vi "main.vi"() -> ()   [LabVIEW 2016]
uses:
  Monochromator/Monochromator.lvclass
  MonoStateFactory/MonoStateFactory.lvclass
  ts_labview_tcp/TCPServer/TCPServer.lvclass
  C:/Users/aanania/Documents/ts_monochromator_windows/ts_labview_tcp/TCPCommunicator/TCPCommunicator.lvclass
  ts_labview_tcp/TCPComEvents/TCPComEvents.lvclass
  MonoCommunicator/MonoCommunicator.lvclass
  MonoPubSubData/MonoPubSubData.lvclass
  Typedefs/SWStatus.ctl
  Monochromator/Monochromator.lvclass/Monochromator.ctl
  MonoPubSubData/MonoPubSubData.lvclass/MonoPubSubData.ctl
  MonoCommunicator/MonoCommunicator.lvclass/MonoCommunicator.ctl
  ts_labview_tcp/TCPComEvents/TCPComEvents.lvclass/TCPComEvents.ctl
  ts_labview_tcp/TCPCommunicator/TCPCommunicator.lvclass/TCPCommunicator.ctl
  Monochromator/run.vi
  ts_labview_tcp/TCPSettings/TCPSettings.lvclass
  ts_labview_tcp/TCPCommunicator/TCPCommunicator.lvclass
panel:
  in  "Port":u16=50000
  in  "IP":string="127.0.0.1"
  in  "MonoID":string="Mono1"
  in  "Force Init":bool
  in  "UniqueID":string
  # "Mono Init"
  # "TCP Setting"
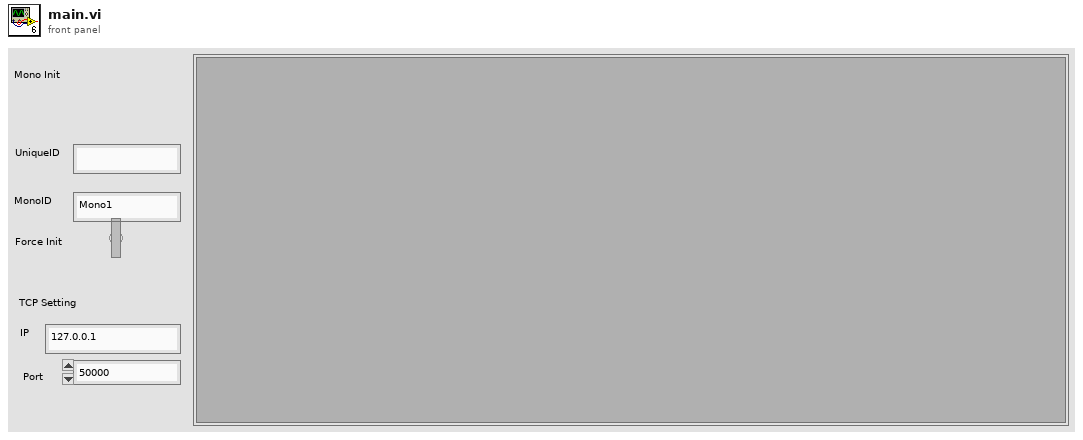
[diagram p1: front panel]
types:
  T1 = typedef "SWStatus.ctl" = enum16{"OfflineState", "ReadyState", "SettingUpState", "FaultState"}
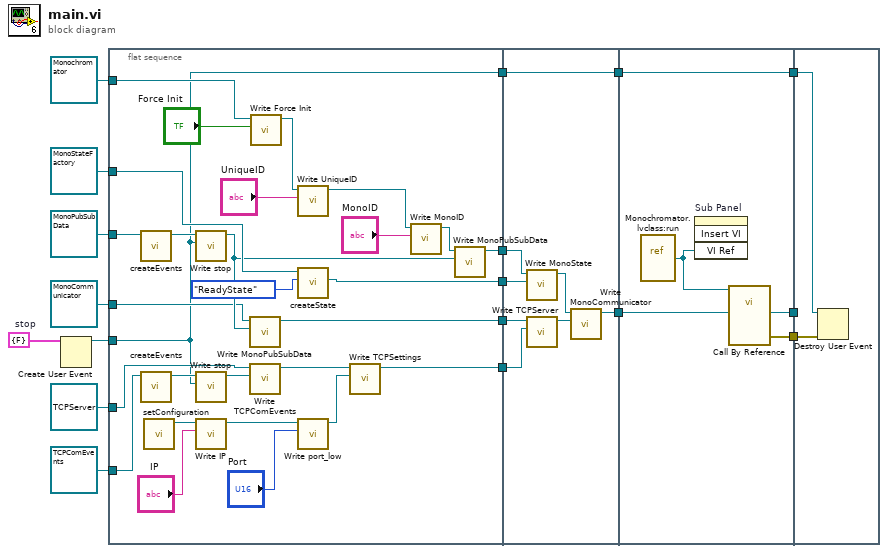
[diagram p0: block diagram]
diagram:
  w12 = cluster{"stop":bool} {"stop"=FALSE}  # stop
  n1 = Create User Event(user event datatype=w12) -> (user event=w11:refnum<user-event>)  [unwired: 1 in, 1 out]
  n2 = flat-sequence {
    tunnel: refnum<class "Monochromator.lvclass"> refnum ("Monochromator.lvclass") -> [w45]
    tunnel: [w32] -> w17
    tunnel: refnum<class "MonoStateFactory.lvclass"> refnum ("MonoStateFactory.lvclass") -> [w42]
    tunnel: [w40] -> w15
    tunnel: refnum<class "TCPComEvents.lvclass"> refnum ("TCPComEvents.lvclass") -> [w39]
    tunnel: refnum<class "TCPServer.lvclass"> refnum ("TCPServer.lvclass") -> [w37]
    tunnel: w11 -> [w27]
    tunnel: [w34] -> w10
    tunnel: refnum<class "MonoPubSubData.lvclass"> refnum ("MonoPubSubData.lvclass") -> [w33]
    tunnel: refnum<class "MonoCommunicator.lvclass"> refnum ("MonoCommunicator.lvclass") -> [w29]
    tunnel: [w28] -> w7
    tunnel: [w27] -> w3
    tunnel: w17 -> [w54]
    tunnel: w15 -> [w53]
    tunnel: w10 -> [w51]
    tunnel: w7 -> [w52]
    tunnel: [w48] -> w6
    tunnel: [w47] -> w4
    tunnel: w3 -> [w47]
    tunnel: w6 -> [w57]
    tunnel: [w59] -> w5
    tunnel: w4 -> [w59]
    tunnel: [w56] -> w2
    tunnel: [w55] -> w1
    tunnel: w5 -> [w61]
    tunnel: w2 -> [_]
    tunnel: w1 -> [w60]
    frame #0 {
      n3 = call "createEvents.vi"("MonoPubSubData in"=w33) -> ("MonoPubSubData out"=w31:refnum<class "MonoPubSubData.lvclass">)  [unwired: 9 in, 1 out]
      n4 = call "createEvents.vi"("TCPComEvents in"=w39) -> ("TCPComEvents out"=w38:refnum<class "TCPComEvents.lvclass">)  [unwired: 9 in, 1 out]
      n5 = call "setConfiguration.vi"() -> ("TCPSettings out"=w23:refnum<class "TCPSettings.lvclass">)  [unwired: 11 in]
      n6 = call "Write stop.vi"("stop"=w27, "MonoPubSubData in"=w31) -> ("MonoPubSubData out"=w30:refnum<class "MonoPubSubData.lvclass">)  [unwired: 8 in, 1 out]
      n7 = call "Write stop.vi"("stop"=w27, "TCPComEvents in"=w38) -> ("TCPComEvents out"=w36:refnum<class "TCPComEvents.lvclass">)  [unwired: 8 in, 1 out]
      n8 = call-dynamic "Write IP.vi"("IP"="IP", "TCPSettings in"=w23) -> ("TCPSettings out"=w21:refnum<class "TCPSettings.lvclass">)  [unwired: 8 in, 1 out]
      n9 = call "Write MonoPubSubData.vi"("MonoPubSubData.lvclass"=w30, "MonoCommunicator in"=w29) -> ("MonoCommunicator out"=w28:refnum<class "MonoCommunicator.lvclass">)  [unwired: 8 in, 1 out]
      n10 = call "Write TCPComEvents.vi"("TCPComEvents.lvclass"=w36, "TCPCommunicator in"=w37) -> ("TCPCommunicator out"=w35:refnum<class "TCPServer.lvclass">)  [unwired: 8 in, 1 out]
      n11 = call "Write Force Init.vi"("Force Init"="Force Init", "Monochromator in"=w45) -> ("Monochromator out"=w44:refnum<class "Monochromator.lvclass">)  [unwired: 8 in, 1 out]
      n12 = call "Write UniqueID.vi"("UniqueID"="UniqueID", "Monochromator in"=w44) -> ("Monochromator out"=w26:refnum<class "Monochromator.lvclass">)  [unwired: 8 in, 1 out]
      n13 = call "createState.vi"("SWStatus"=SWStatus."ReadyState", "MonoStateFactory in"=w42) -> ("MonoState.lvclass"=w40:refnum<class "MonoState.lvclass">)  [unwired: 7 in, 2 out]
      n14 = call-dynamic "Write port_low.vi"("port_low"="Port", "TCPSettings in"=w21) -> ("TCPSettings out"=w19:refnum<class "TCPSettings.lvclass">)  [unwired: 8 in, 1 out]
      n15 = call-dynamic "Write TCPSettings.vi"("TCPSettings.lvclass"=w19, "TCPCommunicator in"=w35) -> ("TCPCommunicator out"=w34:refnum<class "TCPServer.lvclass">)  [unwired: 8 in, 1 out]
      n16 = call "Write MonoID.vi"("MonoID"="MonoID", "Monochromator in"=w26) -> ("Monochromator out"=w25:refnum<class "Monochromator.lvclass">)  [unwired: 8 in, 1 out]
      n17 = call "Write MonoPubSubData.vi"("MonoPubSubData.lvclass"=w30, "Monochromator in"=w25) -> ("Monochromator out"=w32:refnum<class "Monochromator.lvclass">)  [unwired: 8 in, 1 out]
    }
    frame #1 {
      n18 = call "Write MonoState.vi"("MonoState.lvclass"=w53, "Monochromator in"=w54) -> ("Monochromator out"=w50:refnum<class "Monochromator.lvclass">)  [unwired: 8 in, 1 out]
      n19 = call "Write TCPServer.vi"("TCPServer.lvclass"=w51, "MonoCommunicator in"=w52) -> ("MonoCommunicator out"=w49:refnum<class "MonoCommunicator.lvclass">)  [unwired: 8 in, 1 out]
      n20 = call "Write MonoCommunicator.vi"("MonoCommunicator.lvclass"=w49, "Monochromator in"=w50) -> ("Monochromator out"=w48:refnum<class "Monochromator.lvclass">)  [unwired: 8 in, 1 out]
    }
    frame #2 {
      n21 = vi-ref "Monochromator.lvclass:run.vi"() -> (w58:refnum<vi>)
      n22 = invoke on="Sub Panel" class="SubPnl" method="Insert VI"("VI Ref"=w58) -> ()  [unwired: 3 in, 4 out]
      n23 = call-by-ref "?"(reference=w58, "Monochromator in"=w57) -> ("error out"=w55:errorcluster, "Monochromator out"=w56:refnum<class "Monochromator.lvclass">)  [unwired: 10 in, 2 out]
    }
    frame #3 {
      n24 = Destroy User Event(user event=w61, error in=w60) -> ()  [unwired: 1 out]
    }
  }
